vi "FlowMeterStub.vi"(6 "Graph in":cluster{dbl[], dbl[]}, 7 "Index":i32, 8 "error in":errorcluster, 9 "Length":i32=250, 11 "ON":bool) -> (0 "error out":errorcluster, 2 "Values":cluster{dbl[], dbl[]})   [LabVIEW 2012]
uses:
  GlobalVariables/CalibrationState.vi
  GlobalVariables/CalibrationVolumes.vi
  GlobalVariables/Samples.vi
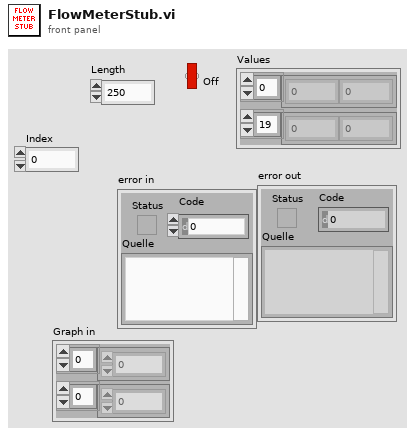
[diagram p1: front panel]
types:
  T1 = cluster{"Pressure":cluster{"TimeSamples":dbl[], "PressureSamples":dbl[]}, "Flow":cluster{"TimeSamples":dbl[], "FlowSamples":dbl[]}}
  T2 = cluster{"CalibrationVolumes":dbl[], "SetName":string}[]
  T3 = cluster{bool, "CalibrationStep":u32, "Volumes":dbl[], "PressureRatios":dbl[], "Weights":bool[]}
  T4 = cluster{"CalibrationVolumes":dbl[], "SetName":string}
  T5 = cluster{"TimeSamples":dbl[], "FlowSamples":dbl[]}
  T6 = cluster{"TimeSamples":dbl[], "PressureSamples":dbl[]}
  T7 = cluster{"Pressure":cluster{"TimeSamples":dbl[], "PressureSamples":dbl[]}, cluster{"TimeSamples":dbl[], "FlowSamples":dbl[]}}
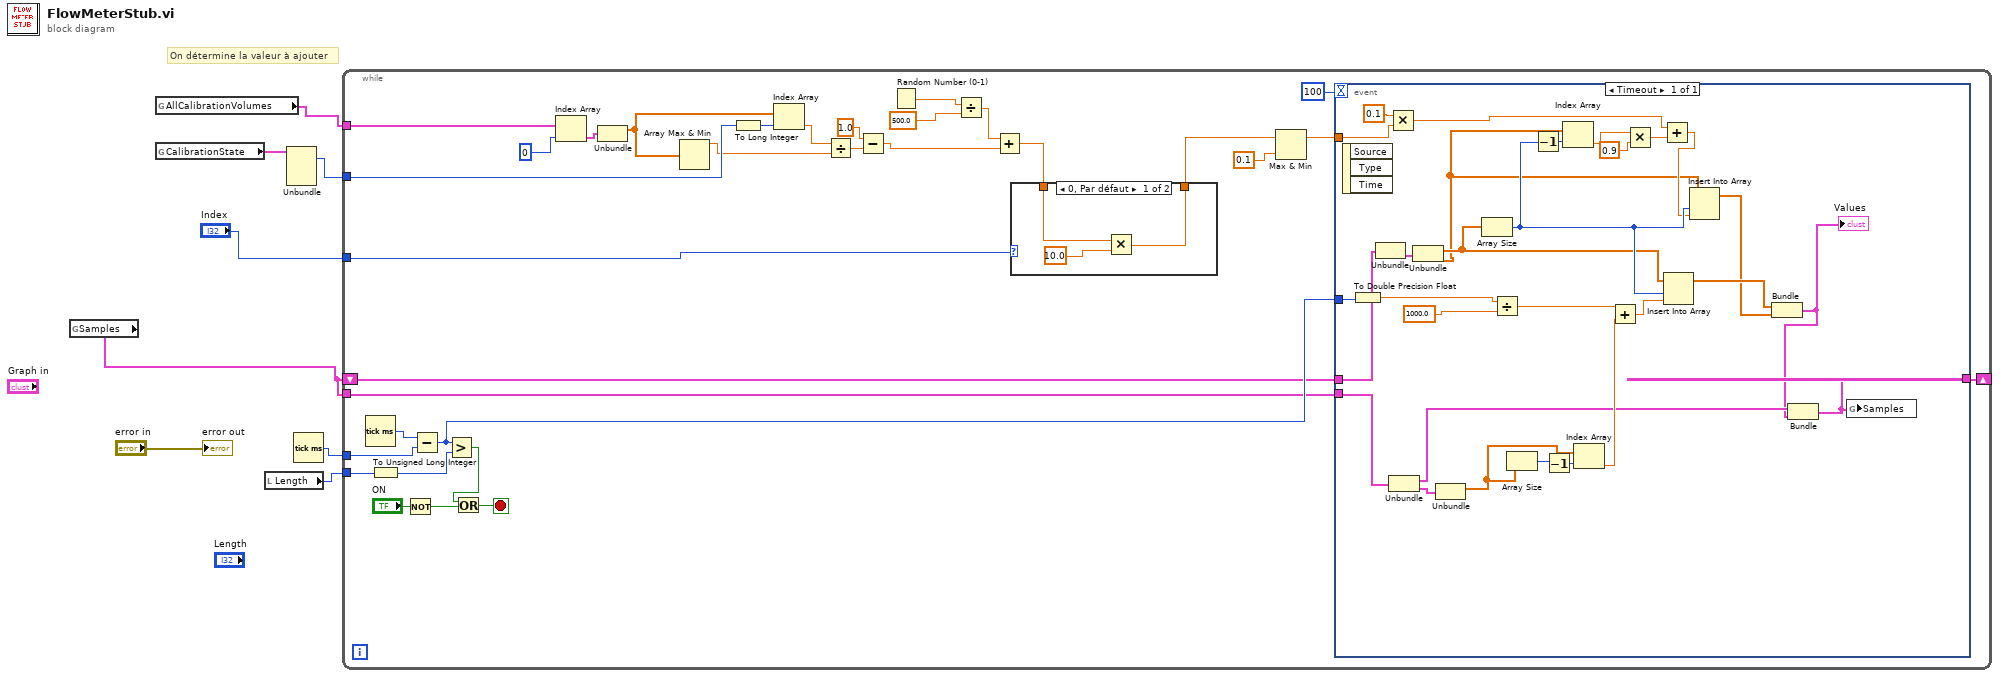
[diagram p0: block diagram]
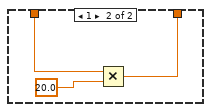
[diagram p2: hidden frame]
diagram:
  # "On détermine la valeur à ajouter"
  n1 = global read "Samples.vi" "Samples"() -> (w2:T1)
  n2 = global read "CalibrationVolumes.vi" "AllCalibrationVolumes"() -> (w4:T2)
  n3 = global read "CalibrationState.vi" "CalibrationState"() -> (w5:T3)
  n4 = local read "Length"() -> (w7:i32)
  n5 = Unbundle(w5) -> ("CalibrationStep"=w3:u32)  [unwired: 4 out]
  n6 = Tick Count (ms)() -> (millisecond timer value=w8:u32)
  n7 = while {
    tunnel: w8 -> [w36]
    tunnel: w7 -> [w31]
    shift-right: [w29] -> _
    shift-left: w2 -> [w32]
    tunnel: w4 -> [w28]
    tunnel: w3 -> [w27]
    tunnel: w2 -> [w18]
    tunnel: "Index" -> [w12]
    stop <- w38 stop-if-true
    n8 = Tick Count (ms)() -> (millisecond timer value=w37:u32)
    n9 = To Unsigned Long Integer(number=w31) -> (unsigned 32bit integer=w30:u32)
    n10 = Not(x="ON") -> (.not. x?=w39:bool)
    n11 = Subtract(x=w37, y=w36) -> (x-y=w33:u32)
    n12 = Greater?(x=w33, y=w30) -> (0:w35:bool)
    n13 = Or(x=w35, y=w39) -> (x .or. y?=w38:bool)
    n14 = Index Array(array=w28, index=0) -> (element=w20:T4)
    n15 = Unbundle(w20) -> ("CalibrationVolumes"=w19:dbl[])  [unwired: 1 out]
    n16 = Array Max & Min(array=w19) -> (max value=w22:dbl)  [unwired: 3 out]
    n17 = To Long Integer(number=w27) -> (32bit integer=w26:i32)
    n18 = Index Array(array=w19, index=w26) -> (element=w23:dbl)
    n19 = Divide(x=w23, y=w22) -> (x/y=w24:dbl)
    n20 = Subtract(x=1.0, y=w24) -> (x-y=w11:dbl)
    n21 = Random Number (0-1)() -> (number: 0 to 1=w16:dbl)
    n22 = Divide(x=w16, y=500.0) -> (x/y=w15:dbl)
    n23 = Add(x=w15, y=w11) -> (x+y=w10:dbl)
    n24 = case shown="0, Par défaut" w12 {
      tunnel: w10 -> [w43 w44]
      tunnel: [w42 w45] -> w9
      frame 0, Default {
        n25 = Multiply(x=w43, y=10.0) -> (x*y=w42:dbl)
      }
      frame 1 {
        n26 = Multiply(x=w44, y=20.0) -> (x*y=w45:dbl)
      }
    }
    n27 = Max & Min(x=w9, y=0.1) -> (max(x,y)=w14:dbl)  [unwired: 1 out]
    n28 = event shown="[0] Timeout" {
      selector: _ -> [_]
      dyn-events: _ -> [_]
      timeout: 100 -> [_]
      tunnel: w33 -> [w70]
      tunnel: w32 -> [w67]
      tunnel: [w51] -> w29
      tunnel: w14 -> [w61]
      tunnel: w18 -> [w66]
      event Timeout {
        n29 = event-data() -> ()  [unwired: 1 in, 3 out]
        n30 = To Double Precision Float(number=w70) -> (double precision float=w69:dbl)
        n31 = Unbundle(w67) -> ("Flow"=w48:T5)  [unwired: 1 out]
        n32 = Multiply(x=0.1, y=w61) -> (x*y=w59:dbl)
        n33 = Unbundle(w66) -> ("Pressure"=w52:T6, "Flow"=w53:T5)
        n34 = Unbundle(w48) -> ("TimeSamples"=w49:dbl[], "FlowSamples"=w47:dbl[])
        n35 = Unbundle(w53) -> ("TimeSamples"=w54:dbl[])  [unwired: 1 out]
        n36 = Array Size(array=w49) -> (size(s)=w64:i32)
        n37 = Divide(x=w69, y=1000.0) -> (x/y=w72:dbl)
        n38 = Array Size(array=w54) -> (size(s)=w75:i32)
        n39 = Decrement(x=w64) -> (x-1=w65:i32)
        n40 = Decrement(x=w75) -> (x-1=w74:i32)
        n41 = Index Array(array=w47, index=w65) -> (element=w58:dbl)
        n42 = Index Array(array=w54, index=w74) -> (element=w68:dbl)
        n43 = Add(x=w72, y=w68) -> (x+y=w71:dbl)
        n44 = Multiply(x=w58, y=0.9) -> (x*y=w60:dbl)
        n45 = Add(x=w59, y=w60) -> (x+y=w57:dbl)
        n46 = Insert Into Array(array=w49, index=w64, new element=w71) -> (w56:dbl[])
        n47 = Insert Into Array(array=w47, index=w64, new element=w57) -> (w55:dbl[])
        n48 = Bundle("TimeSamples"=w56, "FlowSamples"=w55) -> (w50:T5)  [unwired: 1 in]
        "Values" <- w50
        n49 = Bundle("Pressure"=w52, w50) -> (w51:T7)  [unwired: 1 in]
        n50 = global write "Samples.vi" "Samples"(w51) -> ()
      }
    }
  }
  "error out" <- "error in"
